vi "Pre Launch Init.vi"(11 "NI Force Task in":refnum<class "NI Force Task.lvclass">) -> (0 "error out":errorcluster, 3 "NI Force Task out":refnum<class "NI Force Task.lvclass">)   [LabVIEW 2020, in "NI Force Task.lvlib" / "NI Force Task.lvclass"]
doc: "Initializes the panel actor. Creates the Panel Helper.\n\n----\nPlease see the following web address for additional documentation and tutorial information:\nhttp://www.mooregoodideas.com/mgi-panel-manager/\n\nAuthor: Derek Trepanier\n\nCopyright (c) 2018, Moore Good Ideas, Inc.\n\nAll rights reserved.\n\nRedistribution and use in source and binary forms, with or without modification, are permitted provided that the following conditions are met:\n\n * Redistributions of source code must retain the above copyright notice, this list of conditions and the following disclaimer.\n * Redistributions in binary form must reproduce the above copyright notice, this list of conditions and the following disclaimer in the documentation and/or other materials provided with the distribution.\n * Neither the name of Moore Good Ideas, Inc. nor the names of its contributors may be used to endorse or promote products derived from this software without specific prior written permission.\n\nTHIS SOFTWARE IS PROVIDED BY THE COPYRIGHT HOLDERS AND CONTRIBUTORS \"AS IS\" AND ANY EXPRESS OR IMPLIED WARRANTIES, INCLUDING, BUT NOT LIMITED TO, THE IMPLIED WARRANTIES OF MERCHANTABILITY AND FITNESS FOR A PARTICULAR PURPOSE ARE DISCLAIMED. IN NO EVENT SHALL THE COPYRIGHT OWNER OR CONTRIBUTORS BE LIABLE FOR ANY DIRECT, INDIRECT, INCIDENTAL, SPECIAL, EXEMPLARY, OR CONSEQUENTIAL DAMAGES (INCLUDING, BUT NOT LIMITED TO, PROCUREMENT OF SUBSTITUTE GOODS OR SERVICES; LOSS OF USE, DATA, OR PROFITS; OR BUSINESS INTERRUPTION) HOWEVER CAUSED AND ON ANY THEORY OF LIABILITY, WHETHER IN CONTRACT, STRICT LIABILITY, OR TORT (INCLUDING NEGLIGENCE OR OTHERWISE) ARISING IN ANY WAY OUT OF THE USE OF THIS SOFTWARE, EVEN IF ADVISED OF THE POSSIBILITY OF SUCH DAMAGE."
uses:
  NI Force Task.lvclass
  GUI/NI Tasl df.ctl
  Movement Template df.ctl
  NI Force Task.lvclass/NI Force Task.ctl
  <vilib>/Utility/file.llb/Read Delimited Spreadsheet (DBL).vi
  <vilib>/MGI/Panel Manager/Panel Actor/Panel Actor/Panel Actor.lvclass
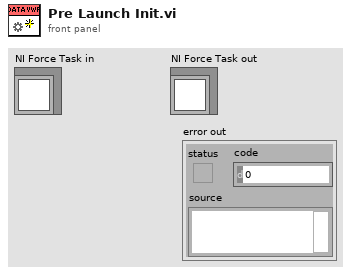
[diagram p1: front panel]
types:
  T1 = typedef "Movement Template df.ctl" = enum16{"Idle", "Update Scanning Template", "Close Helper Loop", "Countdown"}
  T2 = typedef "NI Tasl df.ctl" = enum16{"Idle", "Acquire Force", "Acquire Force and EMG", "Acquire Movement", "Acquire Movement and EMG", "Calibrate Force", "Calibrate Potentiometers", "Collect MVC", "Close Helper Loop", "Collect EMG only", "Countdown"}
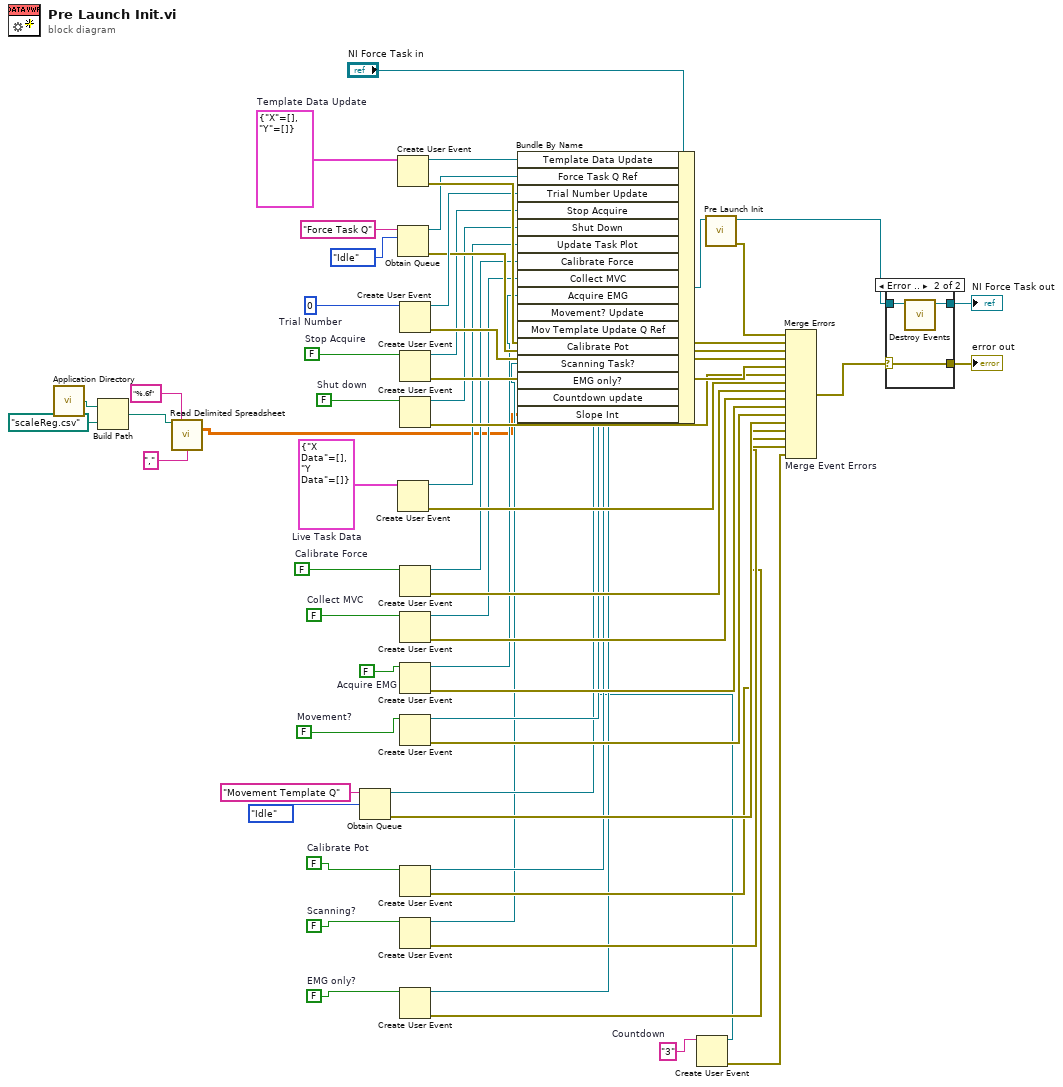
[diagram p0: block diagram]
diagram:
  w9 = "3"  # Countdown
  w12 = FALSE  # EMG only?
  w15 = FALSE  # Scanning?
  w18 = FALSE  # Calibrate Pot
  w25 = FALSE  # Movement?
  w28 = FALSE  # Acquire EMG
  w32 = FALSE  # Collect MVC
  w34 = FALSE  # Calibrate Force
  w47 = 0  # Trial Number
  w39 = cluster{"X Data":dbl[], "Y Data":dbl[]} {"X Data"=[], "Y Data"=[]}  # Live Task Data
  w35 = FALSE  # Shut down
  w36 = FALSE  # Stop Acquire
  w52 = cluster{"X":dbl[], "Y":dbl[]} {"X"=[], "Y"=[]}  # Template Data Update
  n1 = call <vilib>:"Application Directory.vi"() -> ("Application Directory"=w6:path)
  n2 = Build Path(base path=w6, name or relative path=path "scaleReg.csv") -> (appended path=w4:path)
  n3 = call-poly <vilib>:"Read Delimited Spreadsheet.vi"("file path (dialog if empty)"=w4, "format (%.3f)"="%.6f", "delimiter (\\t)"="," ("delimiter (\\t)")) -> ("all rows"=w1:dbl[][])  [unwired: 7 in, 5 out]
  n4 = Obtain Queue(name (unnamed)="Movement Template Q", element data type=Movement_Template_df."Idle") -> (queue out=w20:refnum<queue>, error out=w19:errorcluster)  [unwired: 3 in, 1 out]
  n5 = Create User Event(user event datatype=w52) -> (user event=w51:refnum<user-event>, error out=w60:errorcluster)  [unwired: 1 in]
  n6 = Obtain Queue(name (unnamed)="Force Task Q", element data type=NI_Tasl_df."Idle" ("Enum")) -> (queue out=w48:refnum<queue>, error out=w43:errorcluster)  [unwired: 3 in, 1 out]
  n7 = Create User Event(user event datatype=w39) -> (user event=w38:refnum<user-event>, error out=w37:errorcluster)  [unwired: 1 in]
  n8 = Create User Event(user event datatype=w47) -> (user event=w46:refnum<user-event>, error out=w44:errorcluster)  [unwired: 1 in]
  n9 = Create User Event(user event datatype=w36) -> (user event=w42:refnum<user-event>, error out=w45:errorcluster)  [unwired: 1 in]
  n10 = Create User Event(user event datatype=w35) -> (user event=w40:refnum<user-event>, error out=w41:errorcluster)  [unwired: 1 in]
  n11 = Create User Event(user event datatype=w34) -> (user event=w30:refnum<user-event>, error out=w33:errorcluster)  [unwired: 1 in]
  n12 = Create User Event(user event datatype=w32) -> (user event=w29:refnum<user-event>, error out=w31:errorcluster)  [unwired: 1 in]
  n13 = Create User Event(user event datatype=w28) -> (user event=w27:refnum<user-event>, error out=w26:errorcluster)  [unwired: 1 in]
  n14 = Create User Event(user event datatype=w25) -> (user event=w23:refnum<user-event>, error out=w24:errorcluster)  [unwired: 1 in]
  n15 = Create User Event(user event datatype=w18) -> (user event=w17:refnum<user-event>, error out=w16:errorcluster)  [unwired: 1 in]
  n16 = Create User Event(user event datatype=w15) -> (user event=w13:refnum<user-event>, error out=w14:errorcluster)  [unwired: 1 in]
  n17 = Create User Event(user event datatype=w12) -> (user event=w10:refnum<user-event>, error out=w11:errorcluster)  [unwired: 1 in]
  n18 = Create User Event(user event datatype=w9) -> (user event=w7:refnum<user-event>, error out=w8:errorcluster)  [unwired: 1 in]
  n19 = Bundle By Name(cluster="NI Force Task in", "Template Data Update"=w51, "Force Task Q Ref"=w48, "Trial Number Update"=w46, "Stop Acquire"=w42, "Shut Down"=w40, "Update Task Plot"=w38, "Calibrate Force"=w30, "Collect MVC"=w29, "Acquire EMG"=w27, "Movement? Update"=w23, "Mov Template Update Q Ref"=w20, "Calibrate Pot"=w17, "Scanning Task?"=w13, "EMG only?"=w10, "Countdown update"=w7, "Slope Int"=w1) -> (w58:refnum<class "NI Force Task.lvclass">)
  n20 = call-parent "Pre Launch Init.vi"("Panel Actor in"=w58) -> ("error out"=w57:errorcluster, "Panel Actor out"=w56:refnum<class "NI Force Task.lvclass">)  [unwired: 9 in]
  n21 = Merge Errors "Merge Event Errors"(w57, w60, w43, w44, w45, w41, w37, w33, w31, w26, w24, w19, w16, w14, w11, w8) -> (w54:errorcluster)
  n22 = case shown="Error .." w54 {
    selector: w54 -> [w61 w63]
    tunnel: w56 -> [w62 w65]
    tunnel: [w62 w64] -> w55
    tunnel: [w61 w63] -> w53
    frame No Error {
    }
    frame Error {
      n23 = call "Destroy Events.vi"("NI Force Task in"=w65) -> ("NI Force Task out"=w64:refnum<class "NI Force Task.lvclass">)  [unwired: 9 in, 1 out]
    }
  }
  "error out" <- w53
  "NI Force Task out" <- w55
